vi "onCreate.vi"(8 "error in (no error)":errorcluster, 11 "MQTT_Base in":refnum<class "MQTT_Base.lvclass">) -> (0 "error out":errorcluster, 3 "MQTT_Base out":refnum<class "MQTT_Base.lvclass">)   [LabVIEW 2013, in "MQTT Base.lvlib" / "MQTT_Base.lvclass"]
uses:
  MQTT_Base.lvclass
  Request -- cluster.ctl
  <vilib>/LabVIEW Open Source Project/MQTT Control Packets/Control Packets/ControlPacket/ControlPacket.lvclass
  Response -- cluster.ctl
  Subscription/Subscription.lvclass
  <vilib>/LabVIEW Open Source Project/MQTT Control Packets/Control Packets/PUBLISH/PUBLISH.lvclass
  MQTT_Base.lvclass/MQTT_Base.ctl
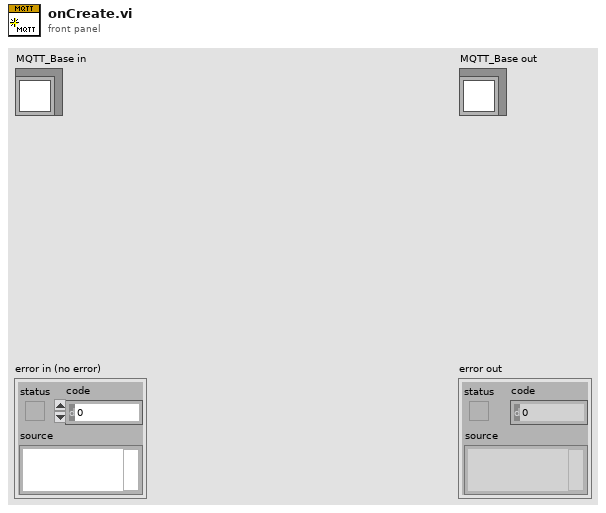
[diagram p1: front panel]
types:
  T1 = typedef "MQTT Base.lvlib/MQTT_Base.lvclass/Request -- cluster.ctl" = cluster{"Packet":refnum<class "ControlPacket.lvclass">, "SessionMailbox":refnum<queue>}
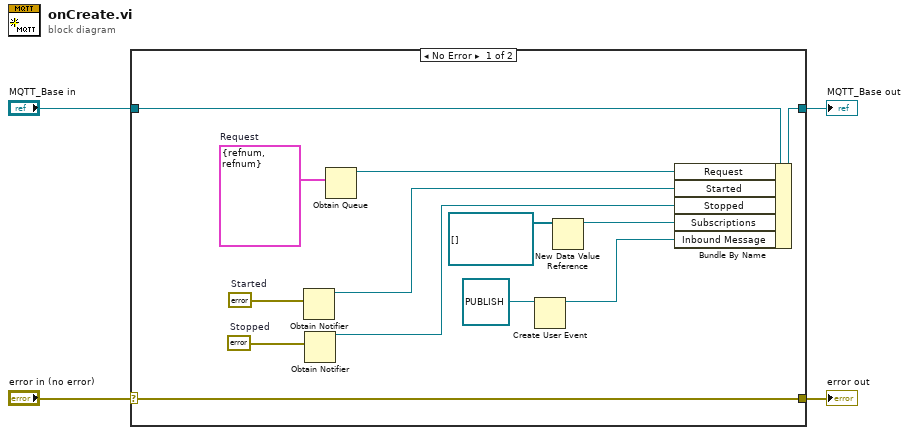
[diagram p0: block diagram]
diagram:
  n1 = case shown="No Error" "error in (no error)" {
    selector: "error in (no error)" -> [w17 w19]
    tunnel: [w17 w19] -> w3
    tunnel: [w11 w18] -> w1
    tunnel: "MQTT_Base in" -> [w12 w18]
    frame No Error {
      w5 = errorcluster {"status"=FALSE, "code"=0, "source"=""}  # Stopped
      w6 = errorcluster {"status"=FALSE, "code"=0, "source"=""}  # Started
      w16 = T1 {"Packet"=refnum, "SessionMailbox"=refnum}  # Request
      n2 = Obtain Notifier(notification data type=w6) -> (notifier out=w14:refnum<notifier>)  [unwired: 3 in, 2 out]
      n3 = Obtain Notifier(notification data type=w5) -> (notifier out=w13:refnum<notifier>)  [unwired: 3 in, 2 out]
      n4 = Obtain Queue(element data type=w16) -> (queue out=w15:refnum<queue>)  [unwired: 4 in, 2 out]
      n5 = Create User Event(user event datatype=refnum<class "PUBLISH.lvclass"> refnum ("PUBLISH.lvclass")) -> (user event=w7:refnum<user-event>)  [unwired: 1 in, 1 out]
      n6 = New Data Value Reference(data value=refnum<class "Subscription.lvclass">[] []) -> (data value reference=w9:refnum<data-value>)  [unwired: 1 in, 1 out]
      n7 = Bundle By Name(cluster=w12, "Request"=w15, "Started"=w14, "Stopped"=w13, "Subscriptions"=w9, "Inbound Message"=w7) -> (w11:refnum<class "MQTT_Base.lvclass">)
    }
    frame Error {
    }
  }
  "error out" <- w3
  "MQTT_Base out" <- w1
